vi "SairDaParede.vi"(10 "Parede":T6(ring), 11 "Robot in":T1) -> (3 "Cluster de saída":T1)   [LabVIEW 2018]
doc: "Função que lida com o atacante quando no estado \"Sair da parede\"."
uses:
  Core/AI Robot.ctl
  Intel/Functions Enum.ctl
  Intel/AttackerStates.ctl
  Path Planning/RRT/PathDests.ctl
  Path Planning/RRT/PathDest.ctl
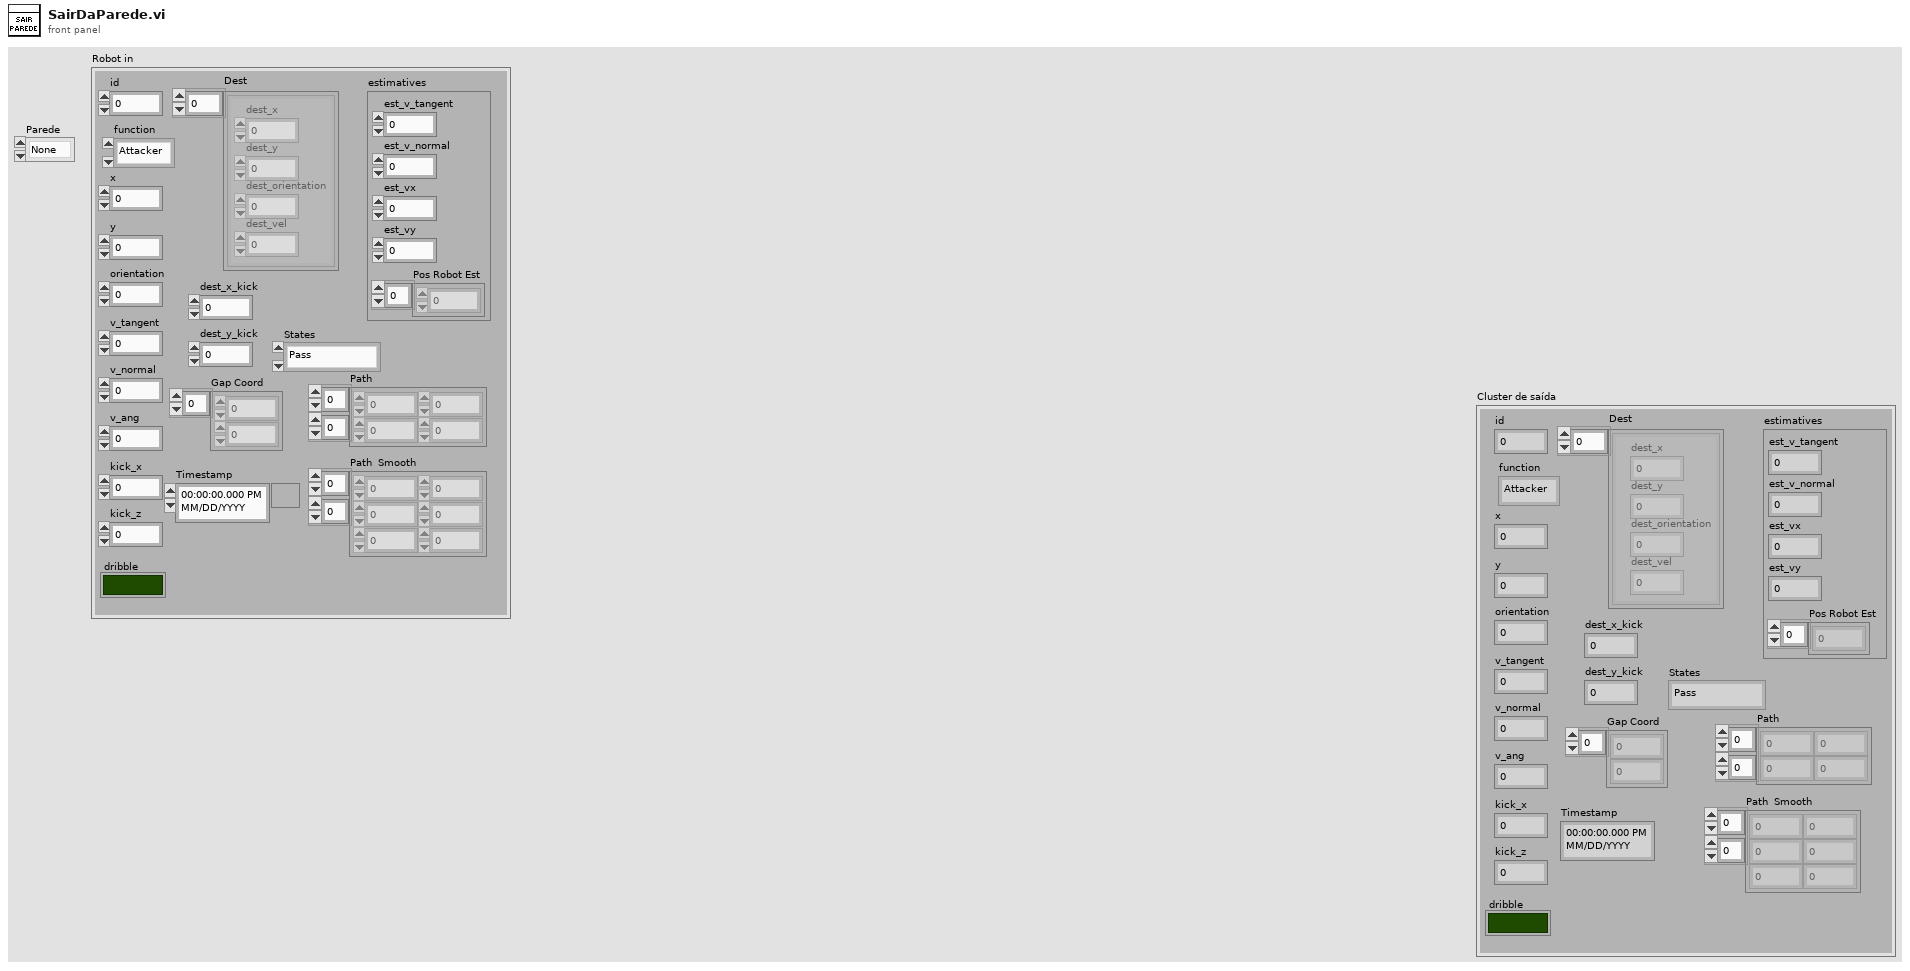
[diagram p1: front panel]
types:
  T1 = typedef "AI Robot.ctl" = cluster{"id":u32, "function":T2, "x":dbl, "y":dbl, "orientation":dbl, "v_tangent":dbl, "v_normal":dbl, "v_ang":dbl, "kick_x":dbl, "kick_z":dbl, "dribble":bool, "Timestamp":timestamp, "estimatives":cluster{"est_v_tangent":dbl, "est_v_normal":dbl, "est_vx":dbl, "est_vy":dbl, "Pos Robot Est":dbl[]}, "dest_x_kick":dbl, "dest_y_kick":dbl, "Gap Coord":dbl[], "States":T3, "Path ":dbl[][], "Path  Smooth":dbl[][], "Dest":T4}
  T2 = typedef "Functions Enum.ctl" = enum16{"Attacker", "Goalie", "Defender", "Striker", "Goto 0", "Dummy", "Kicker", "ZigZag"}
  T3 = typedef "AttackerStates.ctl" = enum16{"Pass", "GoToTangent", "BallGetting", "GoToKick", "Rotate anti-clockwise", "Rotate Clockwise", ""}
  T4 = typedef "PathDests.ctl" = T5[]
  T5 = typedef "PathDest.ctl" = cluster{"dest_x":dbl, "dest_y":dbl, "dest_orientation":dbl, "dest_vel":dbl}
  T6 = enum16{"None", "Frente", "Trás", "Cima", "Baixo"}
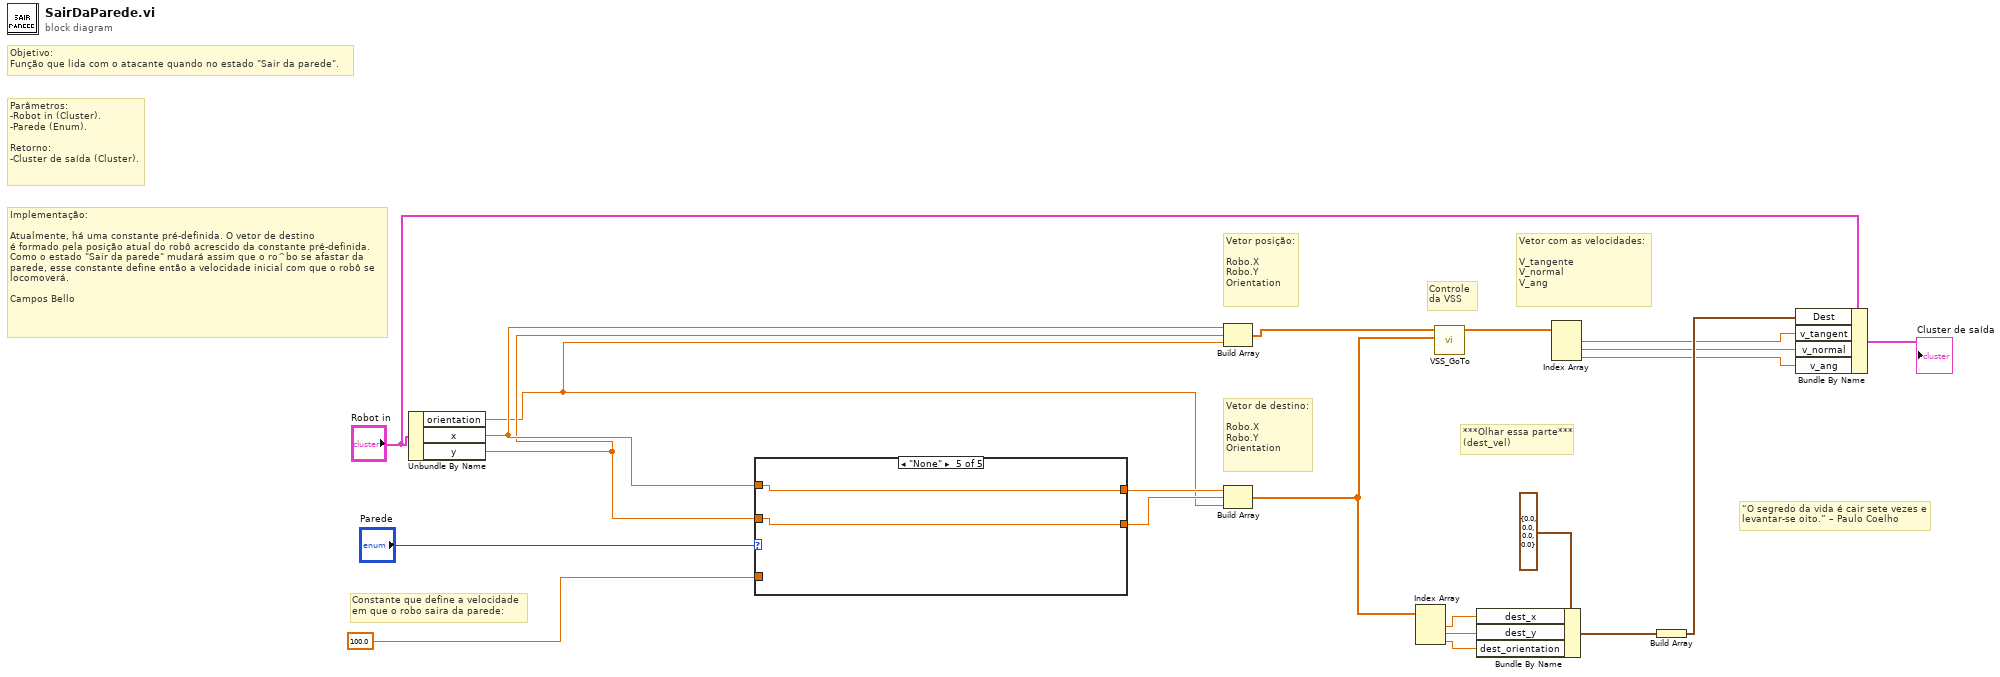
[diagram p0: block diagram]
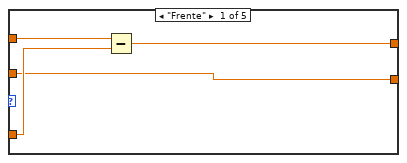
[diagram p2: hidden frame]
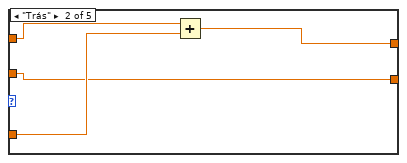
[diagram p3: hidden frame]
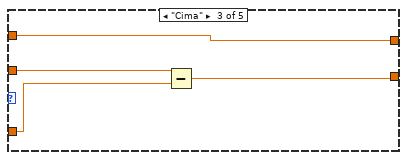
[diagram p4: hidden frame]
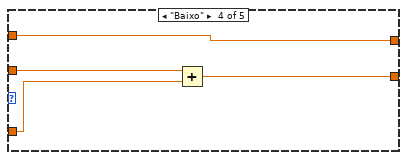
[diagram p5: hidden frame]
diagram:
  # "Implementação:\n\nAtualmente, há uma constante pré-definida. O vetor de destino\né formado pela posição atual do robô acrescido da constante pré-definida.\nComo o estado \"Sair da parede\" mudará assim que o ro^bo se afastar da\nparede, esse constante define então a velocidade inicial com que o robô se\nlocomoverá.\n\nCampos Bello"
  # "Parâmetros:\n-Robot in (Cluster).\n-Parede (Enum).\n\nRetorno:\n-Cluster de saída (Cluster)."
  # "Objetivo:\nFunção que lida com o atacante quando no estado \"Sair da parede\"."
  # "“O segredo da vida é cair sete vezes e\nlevantar-se oito.” – Paulo Coelho"
  # "***Olhar essa parte***\n(dest_vel)"
  # "Controle \nda VSS"
  # "Vetor com as velocidades:\n\nV_tangente\nV_normal\nV_ang"
  # "Vetor posição:\n\nRobo.X\nRobo.Y\nOrientation"
  # "Vetor de destino:\n\nRobo.X\nRobo.Y\nOrientation"
  # "Constante que define a velocidade\nem que o robo saira da parede:"
  n1 = Unbundle By Name("Robot in") -> ("orientation"=w15:dbl, "x"=w17:dbl, "y"=w16:dbl)
  n2 = case shown="\"None\"" "Parede" {
    tunnel: 100.0 -> [w24 w28 w32 w36 _]
    tunnel: w17 -> [w25 w29 w31 w34 w39]
    tunnel: w16 -> [w22 w26 w33 w37 w38]
    tunnel: [w23 w27 w31 w34 w39] -> w19
    tunnel: [w22 w26 w30 w35 w38] -> w18
    frame "Frente" {
      n3 = Subtract(x=w25, y=w24) -> (x-y=w23:dbl)
    }
    frame "Trás" {
      n4 = Add(x=w29, y=w28) -> (x+y=w27:dbl)
    }
    frame "Cima" {
      n5 = Subtract(x=w33, y=w32) -> (x-y=w30:dbl)
    }
    frame "Baixo" {
      n6 = Add(x=w37, y=w36) -> (x+y=w35:dbl)
    }
    frame "None" {
    }
  }
  n7 = Build Array(w17, w16, w15) -> (w13:dbl[])
  n8 = Build Array(w19, w18, w15) -> (w8:dbl[])
  n9 = Index Array(array=w8) -> (element #1=w12:dbl, element #2=w11:dbl, element #3=w10:dbl)  [unwired: 3 in]
  n10 = call "VSS_GoTo.vi"("SetPoint"=w8, "Position"=w13) -> ("Output Vel"=w14:dbl[])  [unwired: 9 in]
  n11 = Bundle By Name(cluster=T5 {"dest_x"=0.0, "dest_y"=0.0, "dest_orientation"=0.0, "dest_vel"=0.0} ("element"), "dest_x"=w12, "dest_y"=w11, "dest_orientation"=w10) -> (w9:T5)
  n12 = Index Array(array=w14) -> (element #1=w3:dbl, element #2=w2:dbl, element #3=w1:dbl)  [unwired: 3 in]
  n13 = Build Array(w9) -> (w4:T5[])
  n14 = Bundle By Name(cluster="Robot in", "Dest"=w4, "v_tangent"=w3, "v_normal"=w2, "v_ang"=w1) -> (→"Cluster de saída":T1)
